vi "Generate LabVIEW Error from Errno.vi"(8 "error in (no error)":errorcluster, 11 "errno":i32) -> (0 "error out":errorcluster)   [LabVIEW 2013, in "Linux Errno.lvlib"]
doc: "This VI receives a return value (errno) from a Linux system function and translates the errno code to a reserved error code range for LabVIEW. If errno indicates an error occurred (errno > 0), a LabVIEW error will be generated."
uses:
  Linux Errno.lvlib
  Controls/errno.ctl
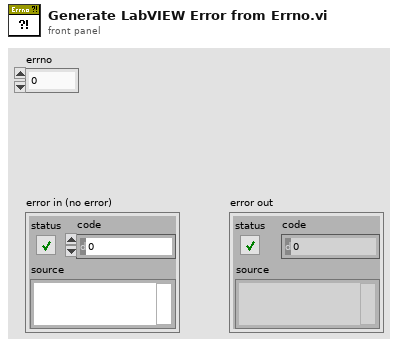
[diagram p1: front panel]
types:
  T1 = typedef "Linux Errno.lvlib/errno.ctl" = enum16{"NONE", "EPERM", "ENOENT", "ESRCH", "EINTR", "EIO", "ENXIO", "E2BIG", "ENOEXEC", "EBADF", "ECHILD", "EAGAIN", "ENOMEM", "EACCES", "EFAULT", "ENOTBLK", "EBUSY", "EEXIST", "EXDEV", "ENODEV", "ENOTDIR", "EISDIR", "EINVAL", "ENFILE", "EMFILE", "ENOTTY", "ETXTBSY", "EFBIG", "ENOSPC", "ESPIPE", "EROFS", "EMLINK", "EPIPE", "EDOM", "ERANGE", "EDADLK", "ENAMETOOLONG", "ENOLCK", "ENOSYS", "ENOTEMPTY", "ELOOP", "EWOULDBLOCK", "ENOMSG", "EIDRM", "ECHRNG", "EL2NSYNC", "EL3HLT", "EL3RST", "ELNRNG", "EUNATCH", "ENOCSI", "EL2HLT", "EBADE", "EBADR", "EXFULL", "ENOANO", "EBADRQC", "EBADSLT", "EDEADLOCK", "EBFONT", "ENOSTR", "ENODATA", "ETIME", "ENOSR", "ENONET", "ENOPKG", "EREMOTE", "ENOLINK", "EADV", "ESRMNT", "ECOMM", "EPROTO", "EMULTIHOP", "EDOTDOT", "EBADMSG", "EOVERFLOW", "ENOTUNIQ", "EBADFD", "EREMCHG", "ELIBACC", "ELIBBAD", "ELIBSCN", "ELIBMAX", "ELIBEXEC", "ELISEQ", "ERESTART", "ESTRPIPE", "EUSERS", "ENOTSOCK", "EDESTADDRREQ", "EMSGSIZE", "EPROTOTYPE", "ENOPROTOOPT", "EPROTONOSUPPORT", "ESOCKTNOSUPPORT", "EOPNOTSUPP", "EPFNOSUPPORT", "EAFNOSUPPORT", "EADDRINUSE", "EADDRNOTAVAIL", "ENETDOWN", "ENETUNREACH", "ENETRESET", "ECONNABORTED", "ECONNRESET", "ENOBUFS", "EISCONN", "ENOTCONN", "ESHUTDOWN", "ETOOMANYREFS", "ETIMEDOUT", "ECONNREFUSED", "EHOSTDOWN", "EHOSTUNREACH", "EALREADY", "EINPROGRESS", "ESTALE", "EUCLEAN", "ENOTNAM", "ENAVAIL", "EISNAM", "EREMOTEIO", "EDQUOT", "ENOMEDIUM", "EMEDIUMTYPE", "ECANCELED", "ENOKEY", "EKEYEXPIRED", "EKEYREVOKED", "EKEYREJECTED", "EOWNERDEAD", "ENOTRECOVERABLE"}
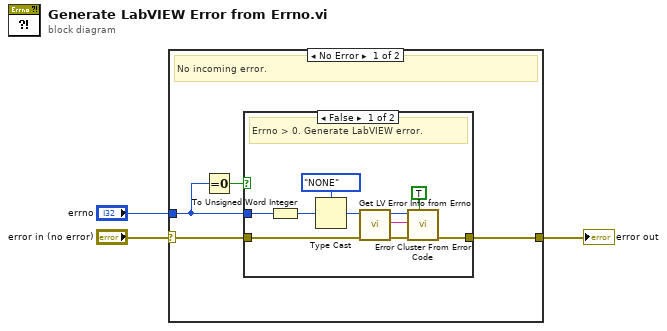
[diagram p0: block diagram]
diagram:
  n1 = case shown="No Error" "error in (no error)" {
    selector: "error in (no error)" -> [w6 w19]
    tunnel: [w5 w19] -> w2
    tunnel: "errno" -> [w4 _]
    frame No Error {
      # "No incoming error."
      n2 = Equal To 0?(x=w4) -> (x = 0?=w7:bool)
      n3 = case shown="False" w7 {
        tunnel: w6 -> [w17 w18]
        tunnel: [w14 w18] -> w5
        tunnel: w4 -> [w8 _]
        frame False {
          # "Errno > 0. Generate LabVIEW error."
          n4 = To Unsigned Word Integer(number=w8) -> (unsigned 16bit integer=w11:u16)
          n5 = Type Cast(type=errno."NONE" ("errno"), x=w11) -> (*(type *) &x=w9:T1)
          n6 = call "Get LV Error Info from Errno.vi"("error in (no error)"=w17, "errno"=w9) -> ("error out"=w12:errorcluster, "error description"=w13:string, "lv error code"=w15:i32)  [unwired: 7 in]
          n7 = call <vilib>:"Error Cluster From Error Code.vi"("show call chain? (False)"=TRUE, "error in (no error)"=w12, "error message (\"\")"=w13, "error code (0)"=w15) -> ("error out"=w14:errorcluster)  [unwired: 5 in]
        }
        frame True {
          # "Errno = 0. No error."
        }
      }
    }
    frame Error {
      # "Error already present. Pass though."
    }
  }
  "error out" <- w2
